vi "volume.vi"(7 "Track Controls":T1 {"Track 3"."Volume" scale=0.01..10.0; "Track 3"."Pan" scale=0.0..1.0; "Track 2"."Volume" scale=0.01..10.0; "Track 2"."Pan" scale=0.0..1.0; "Track 1"."Volume" scale=0.01..10.0; "Track 1"."Pan" scale=0.0..1.0; "Track 0"."Volume" scale=0.01..10.0; "Track 0"."Pan" scale=0.0..1.0}, 8 "error in (no error)":errorcluster, 10 "4-Track Audio in":T3) -> (0 "error out":errorcluster, 2 "4-Track Audio out":T3)   [LabVIEW 2014]
uses:
  Controls/4 Track Audio.ctl
  Controls/Audio In.ctl
  Controls/Track Controls.ctl
  Controls/Track Volume Settings.ctl
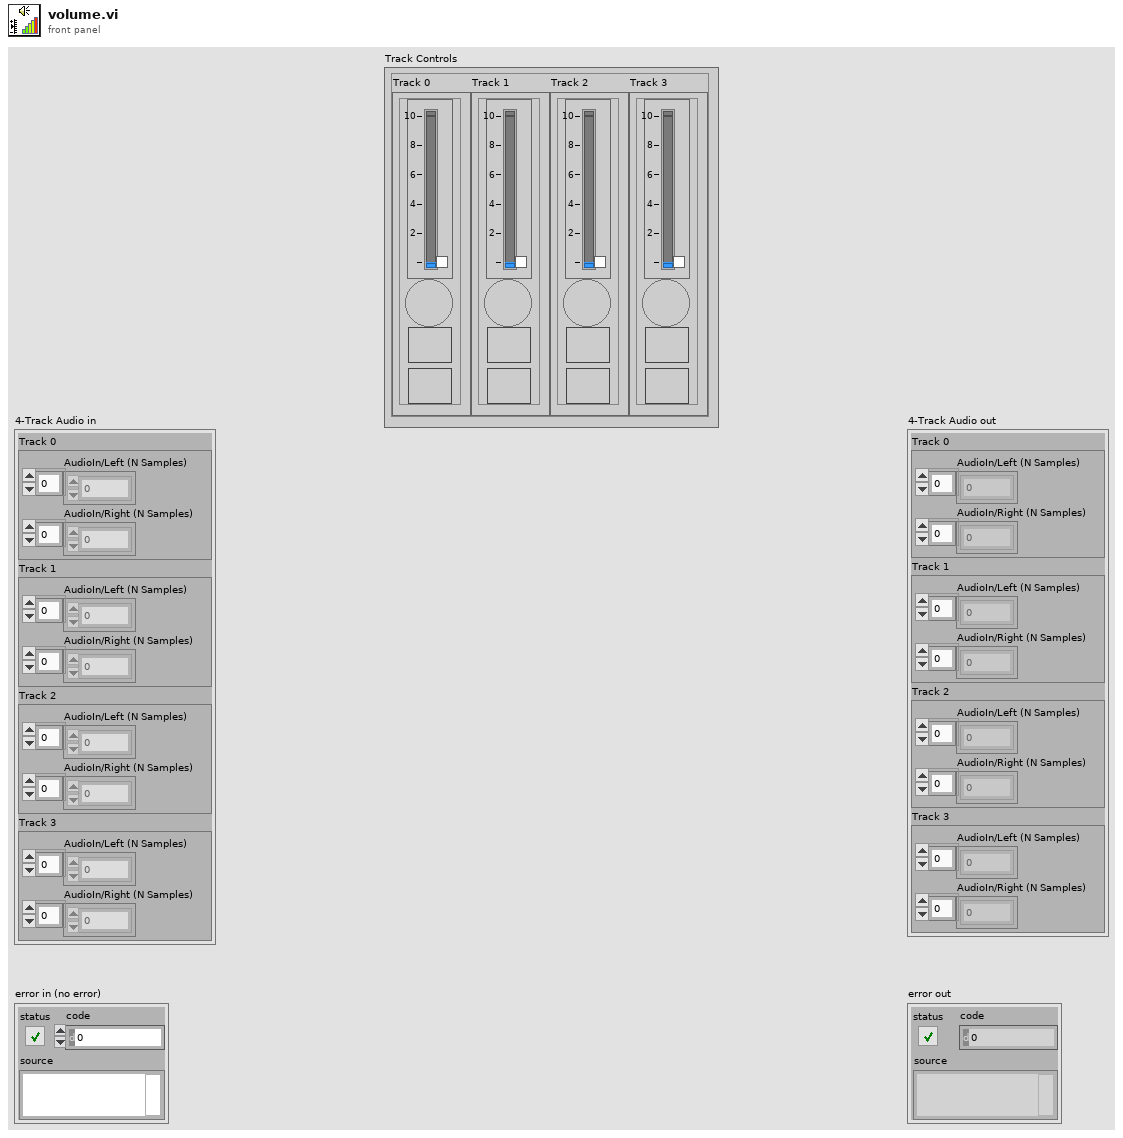
[diagram p1: front panel]
types:
  T1 = typedef "Track Controls.ctl" = cluster{"Track 0":T2, "Track 1":T2, "Track 2":T2, "Track 3":T2}
  T2 = typedef "Track Volume Settings.ctl" = cluster{"Volume":dbl, "Pan":dbl, "Record":bool, "FX":bool}
  T3 = typedef "4 Track Audio.ctl" = cluster{"Track 0":T4, "Track 1":T4, "Track 2":T4, "Track 3":T4}
  T4 = typedef "Audio In.ctl" = cluster{"AudioIn/Left (N Samples)":i16[], "AudioIn/Right (N Samples)":i16[]}
  T5 = cluster{"AudioIn/Left (N Samples)":dbl[], "AudioIn/Right (N Samples)":dbl[]}
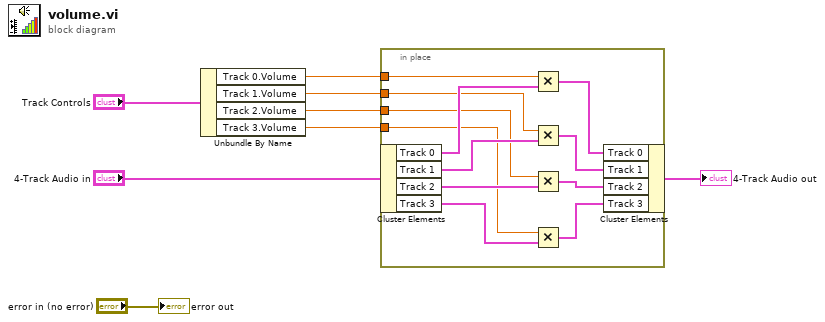
[diagram p0: block diagram]
diagram:
  n1 = Unbundle By Name("Track Controls") -> ("Track 0.Volume"=w5:dbl, "Track 1.Volume"=w4:dbl, "Track 2.Volume"=w3:dbl, "Track 3.Volume"=w2:dbl)
  n2 = in-place {
    in-place-border: w5 -> [w19]
    in-place-border: w4 -> [w15]
    in-place-border: w3 -> [w14]
    in-place-border: w2 -> [w13]
    n3 = in-place-cluster #1("4-Track Audio in") -> ("Track 0"=w20:T4, "Track 1"=w18:T4, "Track 2"=w17:T4, "Track 3"=w16:T4)
    n4 = Multiply(x=w19, y=w20) -> (x*y=w12:T5)
    n5 = Multiply(x=w15, y=w18) -> (x*y=w11:T5)
    n6 = Multiply(x=w14, y=w17) -> (x*y=w10:T5)
    n7 = Multiply(x=w13, y=w16) -> (x*y=w9:T5)
    n8 = in-place-cluster #1("Track 0"=w12, "Track 1"=w11, "Track 2"=w10, "Track 3"=w9) -> (→"4-Track Audio out":T3)
  }
  "error out" <- "error in (no error)"
